vi "newValueGF.vi"(9 "newValue":string, 10 "control":enum16{"read", "write"}(ring)) -> (1 "newValue out":string)   [LabVIEW 2009, in "Compiler.lvlib"]
uses:
  Compiler.lvlib
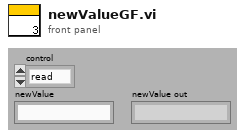
[diagram p1: front panel]
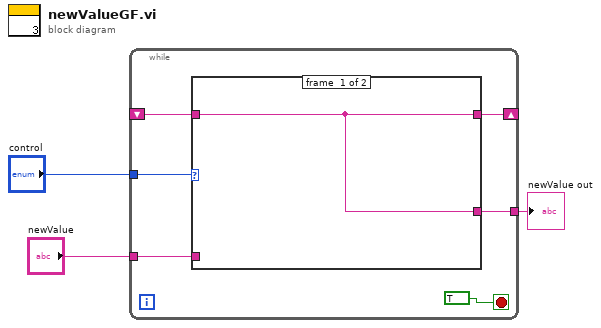
[diagram p0: block diagram]
diagram:
  n1 = while {
    tunnel: "control" -> [w9]
    tunnel: "newValue" -> [w6]
    shift-right: [w7] -> _
    shift-left: _ -> [w5]
    tunnel: [w4] -> w1
    stop <- TRUE stop-if-true
    n2 = case shown="\"read\"" w9 {
      tunnel: [w10 w11] -> w7
      tunnel: w6 -> [_ w11]
      tunnel: w5 -> [w10 _]
      tunnel: [w10 w11] -> w4
      frame #0 {
      }
      frame #1 {
      }
    }
  }
  "newValue out" <- w1
